vi "ApplyLVClassIconOverlayToVIIcon.vi"(0 "LVClassLibrary in":refnum<vi>, 1 "vi refnum in":refnum<vi>, 2 "color":T1, 3 "overlay provided?":bool, 5 "Add ext user layer? (F)":bool, 7 "image data":T1, 9 "255.255.255":u32, 12 "String in":string, 13 "LayerName":string, 14 "new picture":picture) -> (4 "Error code out":i32)   [LabVIEW 2020, in "lv_icon.lvlib"]
uses:
  lv_icon.lvlib
  <vilib>/picture/picture.llb/imagedata.ctl
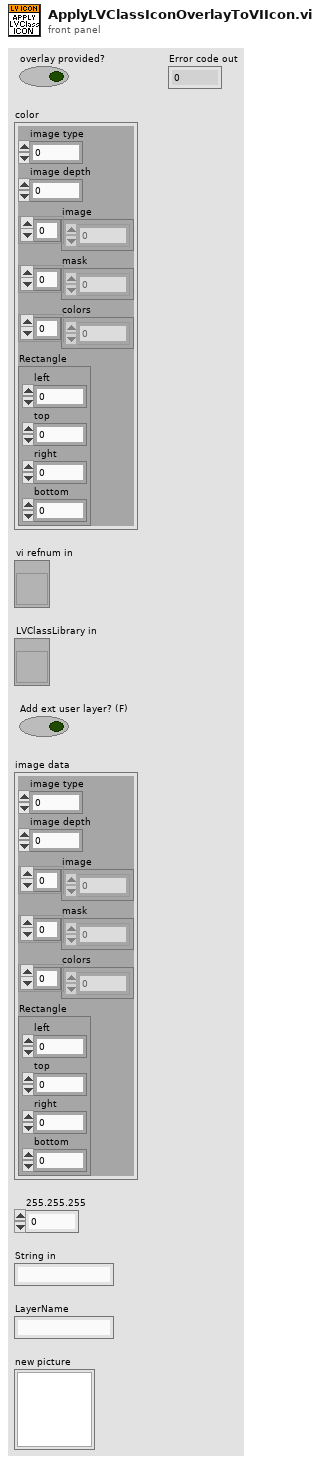
[diagram p1: front panel]
types:
  T1 = typedef "imagedata.ctl" = cluster{"image type":i32, "image depth":i32, "image":u8[], "mask":u8[], "colors":u32[], "Rectangle":cluster{"left":i16, "top":i16, "right":i16, "bottom":i16}}
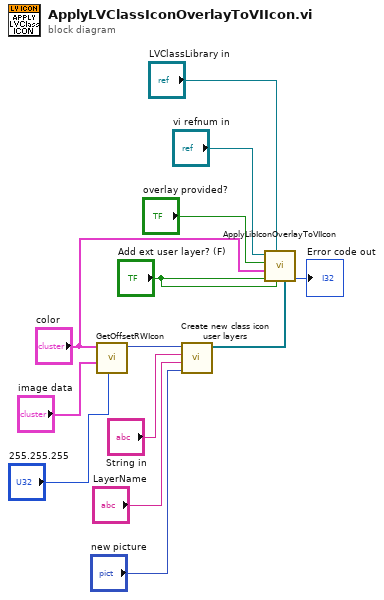
[diagram p0: block diagram]
diagram:
  n1 = call "GetOffsetRWIcon.vi"("Whitespace color"="255.255.255", "R/W overlay"="image data", "Icon"="color") -> ("RW glyph"=w3:picture)  [unwired: 8 in]
  n2 = call "Create new class icon user layers.vi"("new picture"="new picture", "LayerName"="LayerName", "String in"="String in", "RW glyph"=w3) -> ("User Layers"=w12:refnum<class "Layer.lvclass">[])  [unwired: 7 in]
  n3 = call "ApplyLibIconOverlayToVIIcon.vi"("External User Layer"=w12, "Add ext user layer? (F)"="Add ext user layer? (F)", "Lib Refnum"="LVClassLibrary in", "Don't consider curr VI Icon? (F)"="Add ext user layer? (F)", "overlay image"="color", "overlay provided?"="overlay provided?", "VI Refnum"="vi refnum in") -> ("Error code out"=→"Error code out":i32)  [unwired: 4 in]
